vi "Initialize DAQ Assistant.vi"(5 "minimum value":dbl=-5.0 format="%0.2f", 7 "maximum value":dbl=5.0 format="%0.2f", 8 "error in":errorcluster, 9 "rate":dbl=1000.0, 10 "number of samples":i32=100, 11 "physical channels":tag) -> (0 "error out":errorcluster, 3 "task out":refnum<k21>)   [LabVIEW 2022 SP3]
uses:
  <vilib>/DAQmx/create/channels.llb/DAQmx Create Channel (AI-Voltage-Basic).vi
  <vilib>/DAQmx/configure/timing.llb/DAQmx Timing (Sample Clock).vi
  <resource>/objmgr/daqmx.rc
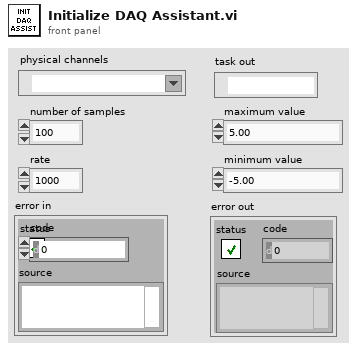
[diagram p1: front panel]
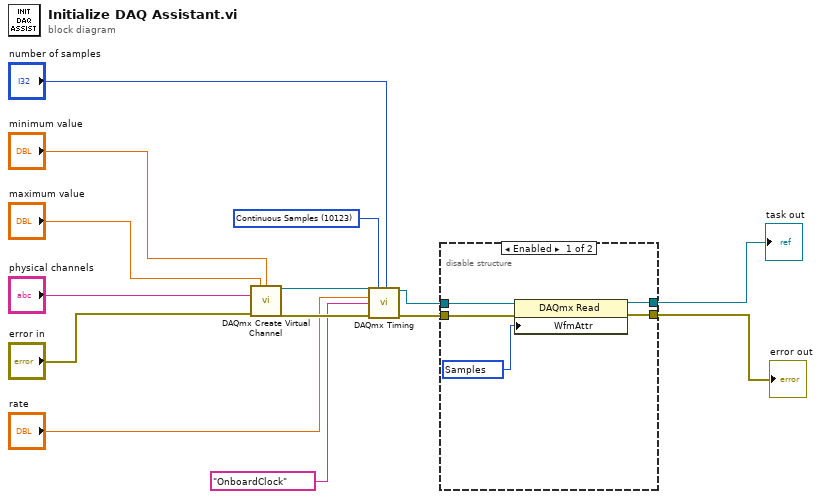
[diagram p0: block diagram]
diagram:
  w12 = 10123 items=["Finite Samples"=10178, "Continuous Samples"=10123, "Hardware Timed Single Point"=12522] ("sample mode")
  n1 = call-poly <vilib>:"DAQmx Create Virtual Channel.vi"("maximum value"="maximum value", "minimum value"="minimum value", "physical channels"="physical channels", "error in"="error in") -> ("task out"=w14:refnum<k21>, "error out"=w13:errorcluster)  [unwired: 10 in]
  n2 = call-poly <vilib>:"DAQmx Timing.vi"("task/channels in"=w14, "sample mode"=w12, "samples per channel"="number of samples", "rate"="rate", "source"=tag "OnboardClock", "error in"=w13) -> ("task out"=w7:refnum<k21>, "error out"=w6:errorcluster)  [unwired: 8 in]
  n3 = disable-structure shown="Enabled" {
    disable-tunnel: w7 -> [w18 w21]
    disable-tunnel: [w17 w21] -> w4
    disable-tunnel: w6 -> [w16 w20]
    disable-tunnel: [w15 w20] -> w3
    frame Enabled {
      w19 = 10287 items=["Samples"=10287, "Samples and Timing"=10140, "Samples, Timing, and Attributes"=10141] ("WfmAttr")
      n4 = property class="DAQmx Read"(reference=w18, error in=w16, "WfmAttr"=w19) -> (reference out=w17:refnum<k21>, error out=w15:errorcluster)
    }
    frame Disabled {
    }
  }
  "error out" <- w3
  "task out" <- w4
